vi "FGV_Vaporizer.vi"(6 "Enum":T2(ring), 8 "error in (no error)":errorcluster caption="Fehler (Eingang, kein Fehler)", 10 "Vaporizer schreiben":T1={"Pumpe Ein/Aus"=0.0, "Wasser / Reagent"=0.0, "Reagent dry / wet"=0.0, "Reagent"=0.0, "min. Temperatur\n160 °C"=160.0, "Solltemperatur"=0.0, "Wasserkonzentration\nSoll"=0.0} {"Reagent" items=["HCI", "HF", "NH3", "Hg", "ppm", "Organik"]; "Reagent dry / wet" items=["wet", "dry"]; "Wasser / Reagent" items=["Wasser", "Reagent"]; "Pumpe Ein/Aus" items=["EIN", "AUS"]}, 11 "Vaporizer lesen":T1={"Pumpe Ein/Aus"=0.0, "Wasser / Reagent"=0.0, "Reagent dry / wet"=0.0, "Reagent"=0.0, "min. Temperatur\n160 °C"=160.0, "Solltemperatur"=0.0, "Wasserkonzentration\nSoll"=0.0} {"Reagent" items=["HCI", "HF", "NH3", "Hg", "ppm", "Organik"]; "Reagent dry / wet" items=["wet", "dry"]; "Wasser / Reagent" items=["Wasser", "Reagent"]; "Pumpe Ein/Aus" items=["EIN", "AUS"]}) -> (0 "error out":errorcluster caption="Fehler (Ausgang)", 1 "Vaporizer %":T1={"Pumpe Ein/Aus"=0.0, "Wasser / Reagent"=0.0, "Reagent dry / wet"=0.0, "Reagent"=0.0, "min. Temperatur\n160 °C"=160.0, "Solltemperatur"=0.0, "Wasserkonzentration\nSoll"=0.0} caption="Vaporizer" {"Reagent" items=["HCI", "HF", "NH3", "Hg", "ppm", "Organik"]; "Reagent dry / wet" items=["wet", "dry"]; "Wasser / Reagent" items=["Wasser", "Reagent"]; "Pumpe Ein/Aus" items=["AUS", "EIN"]}, 2 "Vaporizer_schreiben":T1={"Pumpe Ein/Aus"=0.0, "Wasser / Reagent"=0.0, "Reagent dry / wet"=0.0, "Reagent"=0.0, "min. Temperatur\n160 °C"=160.0, "Solltemperatur"=180.0, "Wasserkonzentration\nSoll"=0.0} caption="Vaüorizer schreiben" {"Reagent" items=["HCI", "HF", "NH3", "Hg", "ppm", "Organik"]; "Reagent dry / wet" items=["wet", "dry"]; "Wasser / Reagent" items=["Wasser", "Reagent"]; "Pumpe Ein/Aus" items=["EIN", "AUS"]}, 3 "Vaporizer_lesen":T1={"Pumpe Ein/Aus"=0.0, "Wasser / Reagent"=0.0, "Reagent dry / wet"=0.0, "Reagent"=0.0, "min. Temperatur\n160 °C"=160.0, "Solltemperatur"=0.0, "Wasserkonzentration\nSoll"=0.0} {"Reagent" items=["HCI", "HF", "NH3", "Hg", "ppm", "Organik"]; "Reagent dry / wet" items=["wet", "dry"]; "Wasser / Reagent" items=["Wasser", "Reagent"]; "Pumpe Ein/Aus" items=["EIN", "AUS"]})   [LabVIEW 2020, in "Linearisierung v2.lvlib" / "Gasteiler.lvlib" / "HovaCal.lvlib"]
uses:
  HovaCal.lvlib
  Vaporizer.ctl
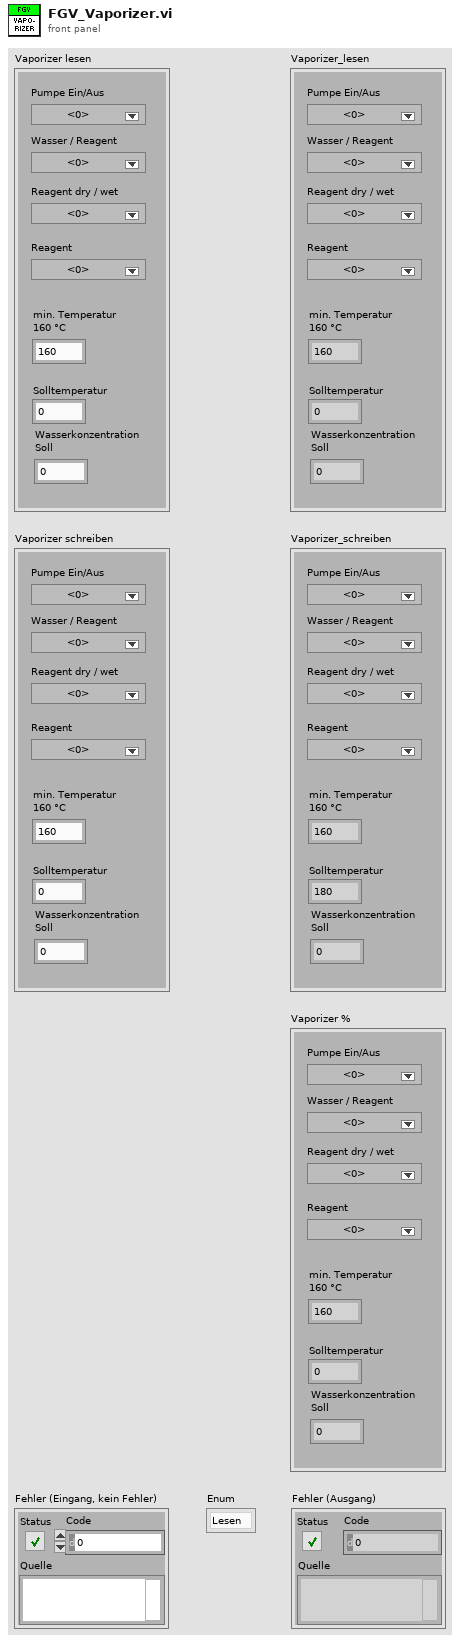
[diagram p1: front panel]
types:
  T1 = typedef "Linearisierung v2.lvlib/Gasteiler.lvlib/HovaCal.lvlib/Vaporizer.ctl" = cluster{"Pumpe Ein/Aus":dbl, "Wasser / Reagent":dbl, "Reagent dry / wet":dbl, "Reagent":dbl, "min. Temperatur\n160 °C":dbl, "Solltemperatur":dbl, "Wasserkonzentration\nSoll":dbl}
  T2 = enum16{"Lesen", "Vaporizer lesen", "Vaporizer schreiben"}
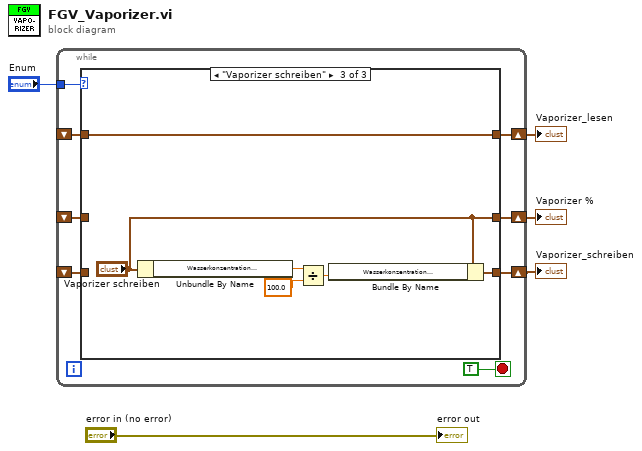
[diagram p0: block diagram]
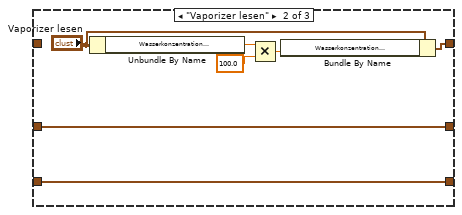
[diagram p3: hidden frame]
diagram:
  n1 = while {
    tunnel: "Enum" -> [w12]
    shift-right: [w11] -> w2
    shift-left: _ -> [w9]
    shift-right: [w10] -> w3
    shift-left: _ -> [w8]
    shift-right: [w7] -> w1
    shift-left: _ -> [w6]
    stop <- TRUE stop-if-true
    n2 = case shown="\"Vaporizer schreiben\"" w12 {
      tunnel: [w16 w18 w29] -> w11
      tunnel: [w15 w23 w25] -> w10
      tunnel: w9 -> [w16 _ w29]
      tunnel: w8 -> [w15 w23 _]
      tunnel: [w14 w17 "Vaporizer schreiben"] -> w7
      tunnel: w6 -> [w14 w17 _]
      frame "Lesen", Default {
      }
      frame "Vaporizer lesen" {
        n3 = Unbundle By Name("Vaporizer lesen") -> ("Wasserkonzentration\nSoll"=w22:dbl)
        n4 = Multiply(x=w22, y=100.0) -> (x*y=w20:dbl)
        n5 = Bundle By Name(cluster="Vaporizer lesen", "Wasserkonzentration\nSoll"=w20) -> (w18:T1)
      }
      frame "Vaporizer schreiben" {
        n6 = Unbundle By Name("Vaporizer schreiben") -> ("Wasserkonzentration\nSoll"=w28:dbl)
        n7 = Divide(x=w28, y=100.0) -> (x/y=w26:dbl)
        n8 = Bundle By Name(cluster="Vaporizer schreiben", "Wasserkonzentration\nSoll"=w26) -> (w25:T1)
      }
    }
  }
  "Vaporizer_lesen" <- w2
  "Vaporizer_schreiben" <- w3
  "Vaporizer %" <- w1
  "error out" <- "error in (no error)"
